vi "Generate Sampling Positions.vi"(5 "Gantry Accel/Decel":dbl=5.0, 7 "Gantry Velocity":dbl=5.0, 9 "Z Range":cluster{"Min":dbl, "Max":dbl, "Increment":dbl}, 10 "Y Range":cluster{"Min":dbl, "Max":dbl, "Increment":dbl}, 11 "X Range":cluster{"Min":dbl, "Max":dbl, "Increment":dbl}) -> (0 "Dimensions":i32[](array[numeric]), 1 "Indices":cluster{i32, i32, i32}[](array[cluster]), 2 "Output":T1[](array[typedef]) {"Z-Position" format="%_7g"; "Y-Position" format="%_7g"; "X-Position" format="%_7g"; "Gantry Velocity" format="%_7g"; "Gantry Accel/Decel" format="%_7g"})   [LabVIEW 2010]
uses:
  Drivers/Motion/Motion_Gantry Position.ctl
panel:
  out "Array Size":i32
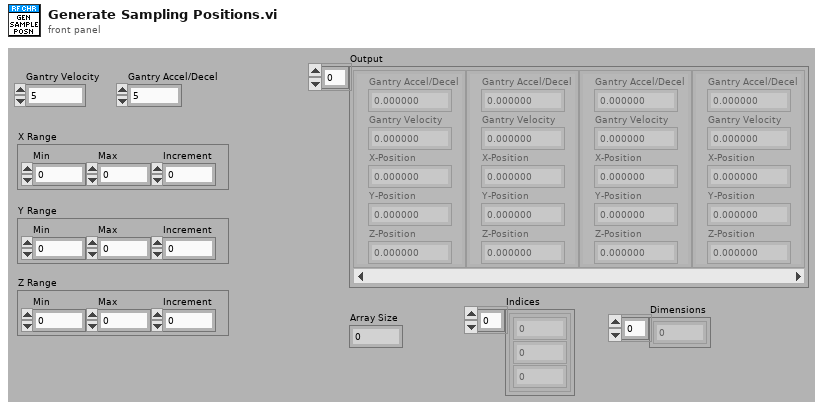
[diagram p1: front panel]
types:
  T1 = typedef "Motion_Gantry Position.ctl" = cluster{"Gantry Accel/Decel":dbl, "Gantry Velocity":dbl, "X-Position":dbl, "Y-Position":dbl, "Z-Position":dbl}
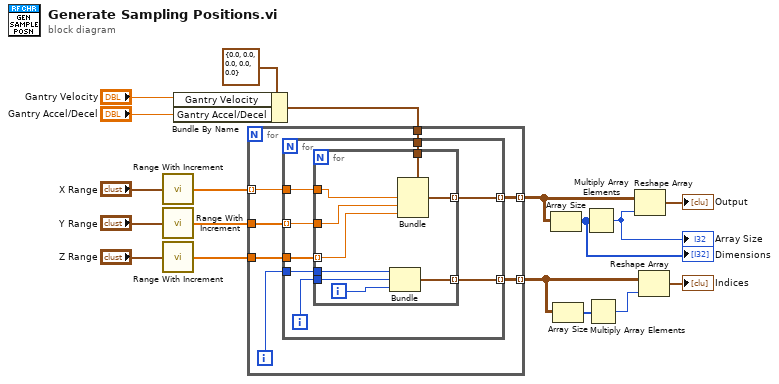
[diagram p0: block diagram]
diagram:
  n1 = call "Range With Increment.vi"("Range"="X Range") -> ("Output Array"=w15:dbl[])
  n2 = call "Range With Increment.vi"("Range"="Y Range") -> ("Output Array"=w14:dbl[])
  n3 = call "Range With Increment.vi"("Range"="Z Range") -> ("Output Array"=w13:dbl[])
  n4 = Bundle By Name(cluster=T1 {"Gantry Accel/Decel"=0.0, "Gantry Velocity"=0.0, "X-Position"=0.0, "Y-Position"=0.0, "Z-Position"=0.0}, "Gantry Velocity"="Gantry Velocity", "Gantry Accel/Decel"="Gantry Accel/Decel") -> (w1:T1)
  n5 = for {
    tunnel: w15 -> [w23] mode=indexing
    tunnel: w14 -> [w25]
    tunnel: w13 -> [w24]
    tunnel: [w22] -> w12 mode=indexing
    tunnel: [w20] -> w8 mode=indexing
    tunnel: w1 -> [w19]
    i -> [w21]
    n6 = for {
      tunnel: w25 -> [w33] mode=indexing
      tunnel: w24 -> [w32]
      tunnel: w23 -> [w31]
      tunnel: [w30] -> w22 mode=indexing
      tunnel: w21 -> [w29]
      tunnel: [w27] -> w20 mode=indexing
      tunnel: w19 -> [w26]
      i -> [w28]
      n7 = for {
        tunnel: w33 -> [w41]
        tunnel: w32 -> [w40] mode=indexing
        tunnel: w31 -> [w42]
        tunnel: [w39] -> w30 mode=indexing
        tunnel: w29 -> [w38]
        tunnel: w28 -> [w37]
        tunnel: [w35] -> w27 mode=indexing
        tunnel: w26 -> [w34]
        i -> [w36]
        n8 = Bundle(w38, w37, w36) -> (w35:cluster{i32, i32, i32})  [unwired: 1 in]
        n9 = Bundle(cluster=w34, "X-Position"=w42, "Y-Position"=w41, "Z-Position"=w40) -> (w39:T1)  [unwired: 2 in]
      }
    }
  }
  n10 = Array Size(array=w12) -> (size(s)=w11:i32[])
  "Dimensions" <- w11
  n11 = Array Size(array=w8) -> (size(s)=w7:i32[])
  n12 = Multiply Array Elements(1:w11) -> (0:w10:i32)
  "Array Size" <- w10
  n13 = Multiply Array Elements(1:w7) -> (0:w6:i32)
  n14 = Reshape Array(w12, w10) -> (→"Output":T1[])
  n15 = Reshape Array(w8, w6) -> (→"Indices":cluster{i32, i32, i32}[])
